vi "write_node.vi"(10 "Signals":dbl) -> ()   [LabVIEW 2014]
panel:
  in  "True/False":bool
  in  "Enable Write":bool=TRUE caption="Enable"
  out "Saving Data":bool
  out "Filename Out":path
  # "Write Node\n\nwrites to excel file"
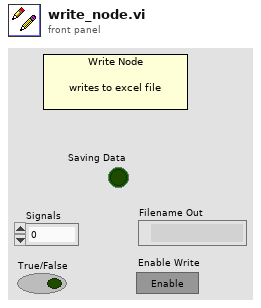
[diagram p1: front panel]
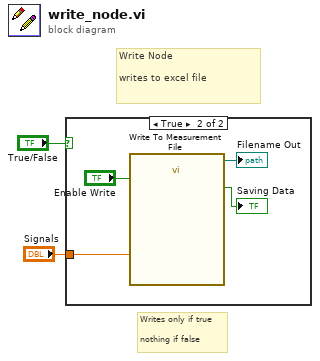
[diagram p0: block diagram]
diagram:
  # "Writes only if true\n\nnothing if false"
  # "Write Node\n\nwrites to excel file"
  n1 = case shown="True" "True/False" {
    tunnel: "Signals" -> [_ w3]
    frame False {
    }
    frame True {
      n2 = call "Write To Measurement File"("Signals"=w3, "Enable"="Enable Write") -> ("Filename Out"=→"Filename Out":path, "Saving Data"=→"Saving Data":bool)  [unwired: 15 in, 1 out]
    }
  }
